vi "Text Width.vi"(10 "String":string, 11 "Font in":refnum<class "Sprite Font.lvclass">) -> (3 "Width":sgl)   [LabVIEW 2021, in "Sprite Font.lvclass"]
uses:
  Sprite Font.lvclass
  Sprite Font.lvclass/Sprite Font.ctl
  Re-use Libraries/Vector 2D/Vector 2D.lvclass/Vector 2D.ctl
  Re-use Libraries/Vector 2D/Vector 2D.lvclass
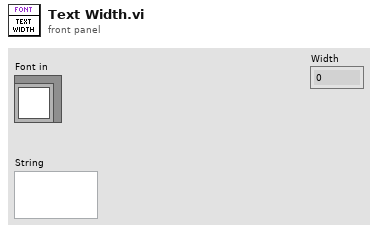
[diagram p1: front panel]
types:
  T1 = typedef "Sprite Font.lvclass/Character.ctl" = cluster{"Texture Name":string, "Size":refnum<class "Vector 2D.lvclass">}
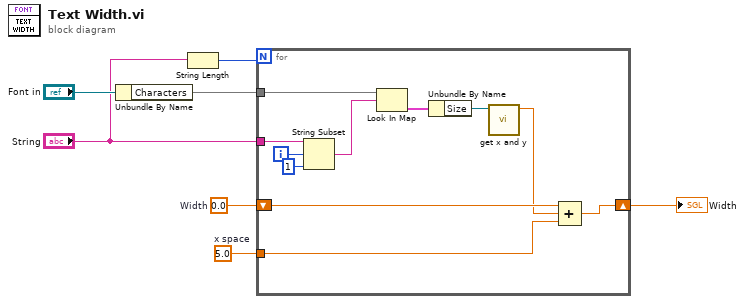
[diagram p0: block diagram]
diagram:
  w2 = sgl 0.0  # Width
  w3 = sgl 5.0  # x space
  n1 = Unbundle By Name("Font in") -> ("Characters"=w6:map{string, T1})
  n2 = String Length(string="String") -> (length=w5:i32)
  n3 = for {
    N: w5 -> [_]
    tunnel: w6 -> [w17]
    shift-right: [w11] -> w1
    shift-left: w2 -> [w10]
    tunnel: "String" -> [w16]
    tunnel: w3 -> [w8]
    i -> [w15]
    n4 = String Subset(string=w16, offset (0)=w15, length (rest)=1 ("length (rest)")) -> (substring=w12:string)
    n5 = Look In Map(map=w17, key=w12) -> (value=w13:T1)  [unwired: 1 in, 1 out]
    n6 = Unbundle By Name(w13) -> ("Size"=w18:refnum<class "Vector 2D.lvclass">)
    n7 = call "get x and y.vi"("Vector 2D in"=w18) -> ("x"=w9:sgl)  [unwired: 9 in, 1 out]
    n8 = Compound Arithmetic op=ADD(w10, w9, w8) -> (w11:sgl)
  }
  "Width" <- w1
